vi "Lock Control in The TopCenter.vi"(6 "offset":cluster{"x":i32, "y":i32}, 8 "error in (no error)":errorcluster, 11 "TabControl in":refnum<vi>) -> (0 "error out":errorcluster)   [LabVIEW 2017]
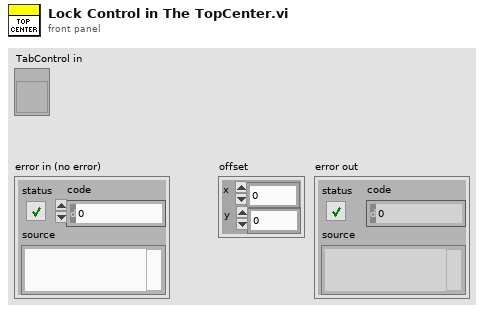
[diagram p1: front panel]
types:
  T1 = typedef "LVBoundsTypeDef.ctl" = cluster{"Width":u32, "Height":u32}
  T2 = typedef "LVPositionTypeDef.ctl" = cluster{"Left":i32, "Top":i32}
  T3 = cluster{"left":i16, "top":i16, "right":i16, "bottom":i16}
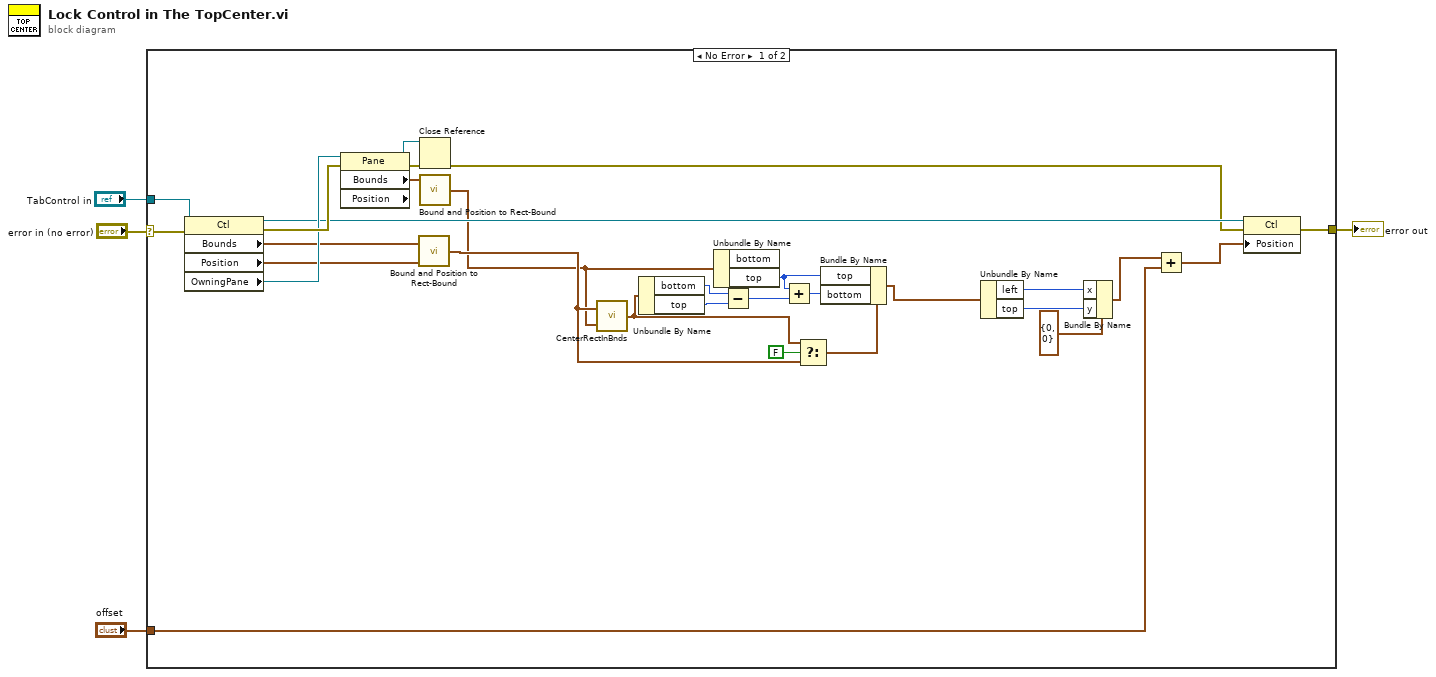
[diagram p0: block diagram]
diagram:
  n1 = case shown="No Error" "error in (no error)" {
    selector: "error in (no error)" -> [w22 w34]
    tunnel: "TabControl in" -> [w24 _]
    tunnel: [w23 w34] -> w3
    tunnel: "offset" -> [w17 _]
    frame No Error {
      n2 = property on="Property Node" class="Ctl"(reference=w24, error in=w22) -> (reference out=w30:refnum<vi>, error out=w32:errorcluster, "Bounds"=w25:T1, "Position"=w26:T2, "OwningPane"=w31:refnum<vi>)
      n3 = property on="Property Node" class="Pane" props=["Bounds", "Position"](reference=w31, error in=w32) -> (reference out=w20:refnum<vi>, error out=w33:errorcluster, "Bounds"=w27:T1)  [unwired: 1 out]
      n4 = call "Bound and Position to Rect-Bound.vi"("Position"=w26, "Bounds"=w25) -> ("Rect Bound"=w29:T3)  [unwired: 3 in]
      n5 = Close Reference(reference=w20, error in (no error)=w33) -> (error out=w21:errorcluster)
      n6 = call "Bound and Position to Rect-Bound.vi"("Bounds"=w27) -> ("Rect Bound"=w28:T3)  [unwired: 4 in]
      n7 = call <vilib>:"CenterRectInBnds.vi"("bounds"=w28, "rect"=w29) -> ("centered rect"=w13:T3)
      n8 = Unbundle By Name(w13) -> ("bottom"=w8:i16, "top"=w9:i16)
      n9 = Unbundle By Name(w28) -> ("top"=w12:i16)  [unwired: 1 out]
      n10 = Subtract(x=w8, y=w9) -> (x-y=w10:i16)
      n11 = Add(x=w12, y=w10) -> (x+y=w11:i16)
      n12 = Select(t=w13, s=FALSE ("centered? (F)"), f=w29) -> (s? t:f=w14:T3)
      n13 = Bundle By Name(cluster=w14, "top"=w12, "bottom"=w11) -> (w19:T3)
      n14 = Unbundle By Name(w19) -> ("left"=w6:i16, "top"=w7:i16)
      n15 = Bundle By Name(cluster=cluster{"x":i32, "y":i32} {"x"=0, "y"=0} ("Point"), "x"=w6, "y"=w7) -> (w18:cluster{"x":i32, "y":i32})
      n16 = Add(x=w18, y=w17) -> (x+y=w16:cluster{"x":i32, "y":i32})
      n17 = property on="Property Node" class="Ctl"(reference=w30, error in=w21, "Position"=w16) -> (error out=w23:errorcluster)  [unwired: 1 out]
    }
    frame Error {
    }
  }
  "error out" <- w3
